vi "LED_voltage_stability.vi"() -> ()   [LabVIEW 2012]
uses:
  <instrlib>/Keithley 2600 Series/Public/Channel.ctl
  <vilib>/Utility/file.llb/Read From Spreadsheet File (DBL).vi
  <vilib>/Utility/file.llb/Write To Spreadsheet File (string).vi
  <vilib>/Utility/file.llb/Write To Spreadsheet File (DBL).vi
  <instrlib>/Keithley 2600 Series/Keithley 2600 Series.lvlib
  <vilib>/Analysis/NI_AALPro.lvlib
  <vilib>/gmath/NI_Gmath.lvlib
panel:
  out "CurDen array":string[](array[string])
  out "power array":string[](array[string])
  out "Power(W)":dbl
  out "DeltaWL":dbl[](array[numeric])
  out "data path":path
  out "DarkSpectrum path":path
  out "Info path":path
  out "AllSpectrum path":path
  out "EQE array":string[](array[string])
  out "LPE array":string[](array[string])
  out "CE array":string[](array[string])
  out "L/L0 array":string[](array[string])
  out "Lum array":string[](array[string])
  out "voltage array":string[](array[string])
  out "current array":string[](array[string])
  out "time array":string[](array[string])
  out "Info3":string
  out "Info2":string
  out "Info1":string
  out "time string":string
  out "date string":string
  out "Status":string
  in  "Tab Control":T1(tab)
  in  "VISA resource name":refnum<visa-resource-name>
  in  "Source Voltage (V)":dbl=2.5 format="%#_5f"
  in  "Current Limit (A)":dbl=1.0 format="%#_5e"
  in  "Integration Time (ms)":dbl=10.0
  in  "Interval (s)":u32=5
  in  "Initial wait (ms)":u32=2000
  in  "Calibration File":path
  in  "Dev_Area (m2)":dbl=3e-06
  in  "WL_high":dbl=785.0
  in  "WL_low":dbl=365.0
  in  "Ratio for auto stop":dbl
  in  "File Path":path
  in  "Auto stop":bool
  in  "Boxcar Width":i32
  in  "Sample description:":string="Please write here..."
  out "Measured Voltage (V)":string
  out "Measured Current (A)":string
  out "WL_2":dbl format="%#_5g"
  out "WL_1":dbl format="%#_5g"
  out "EQE (%)":dbl format="%_3e"
  out "Lum. Pow. Eff. (lm/W)":dbl format="%_3e"
  out "Lum.(cd/m2)":dbl format="%_3e"
  out "Cur. Eff. (cd/A)":dbl format="%_3e"
  out "Lum0":dbl format="%_3e"
  out "Lum/Lum0":dbl format="%_3e"
  out "Time (s)":dbl
  out "Spectra":T2(graph)
  out "Graph":cluster{dbl[], dbl[]}(graph)
  out "Measured_Current(A)":dbl format="%_3e"
  out "Measured_voltage(V)":dbl format="%_3e"
  in  "Ring":i32(ring)=1 items=["L/L0", "Lum", "C.E.", "L.P.E.", "EQE", "Power"]
  out "Maximum Intensity":i32 format="%.2e"
  out "BoxcarWidth":i32
  out "Detector Saturated":bool
  out "All Info":string
  out "VISA resource name out":refnum<visa-resource-name>
  out "error out":errorcluster
  out "x2":i32
  out "x1":i32
  out "Photon_count":dbl
  out "Energy_WL":dbl[](array[numeric])
  out "Candela":dbl
  out "Abs_Irr (W/nm)":dbl[](array[numeric])
  out "Dark_spectrum":dbl[](array[numeric])
  out "Keithley":bool
  out "Spectrometer":bool
  out "Current density (mA/cm2)":dbl
  out "Iso. Coef. itpl":dbl[](array[numeric]) format="%_6g"
  out "WL itpl":dbl[](array[numeric]) format="%_6g"
  out "EyeRespCoef.":dbl[](array[numeric])
  out "WL_EyeResp":dbl[](array[numeric])
  out "WL_cal":dbl[](array[numeric])
  out "cal_CountsToAbsIrr":dbl[](array[numeric])
  in  "Start":bool
  in  "stop":bool
  out "Measured_Spectrum":dbl[](array[numeric])
  out "Wrapper Out":u64
  out "WL_spectrometer":dbl[](array[numeric])
  out "Number of Spectrometers":i32
  out "Node Out":string
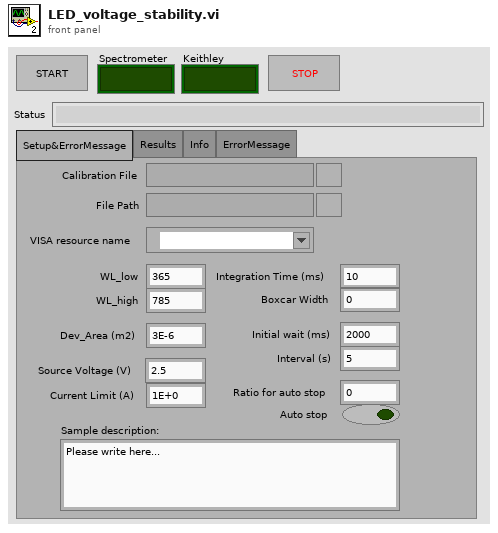
[diagram p1: front panel]
types:
  T1 = enum32{"Setup&ErrorMessage", "Results", "Info", "ErrorMessage"}
  T2 = cluster{"WL_spectrometer":dbl[], "Dark_spectrum":dbl[]}
  T3 = enum32{"Current", "Voltage", "IV", "Resistance", "Power"}
  T4 = typedef "Keithley 2600 Series.lvlib/Channel.ctl" = enum32{"Channel A", "Channel B"}
  T5 = cluster{"WL_spectrometer":dbl[], "Measured_Spectrum":dbl[]}
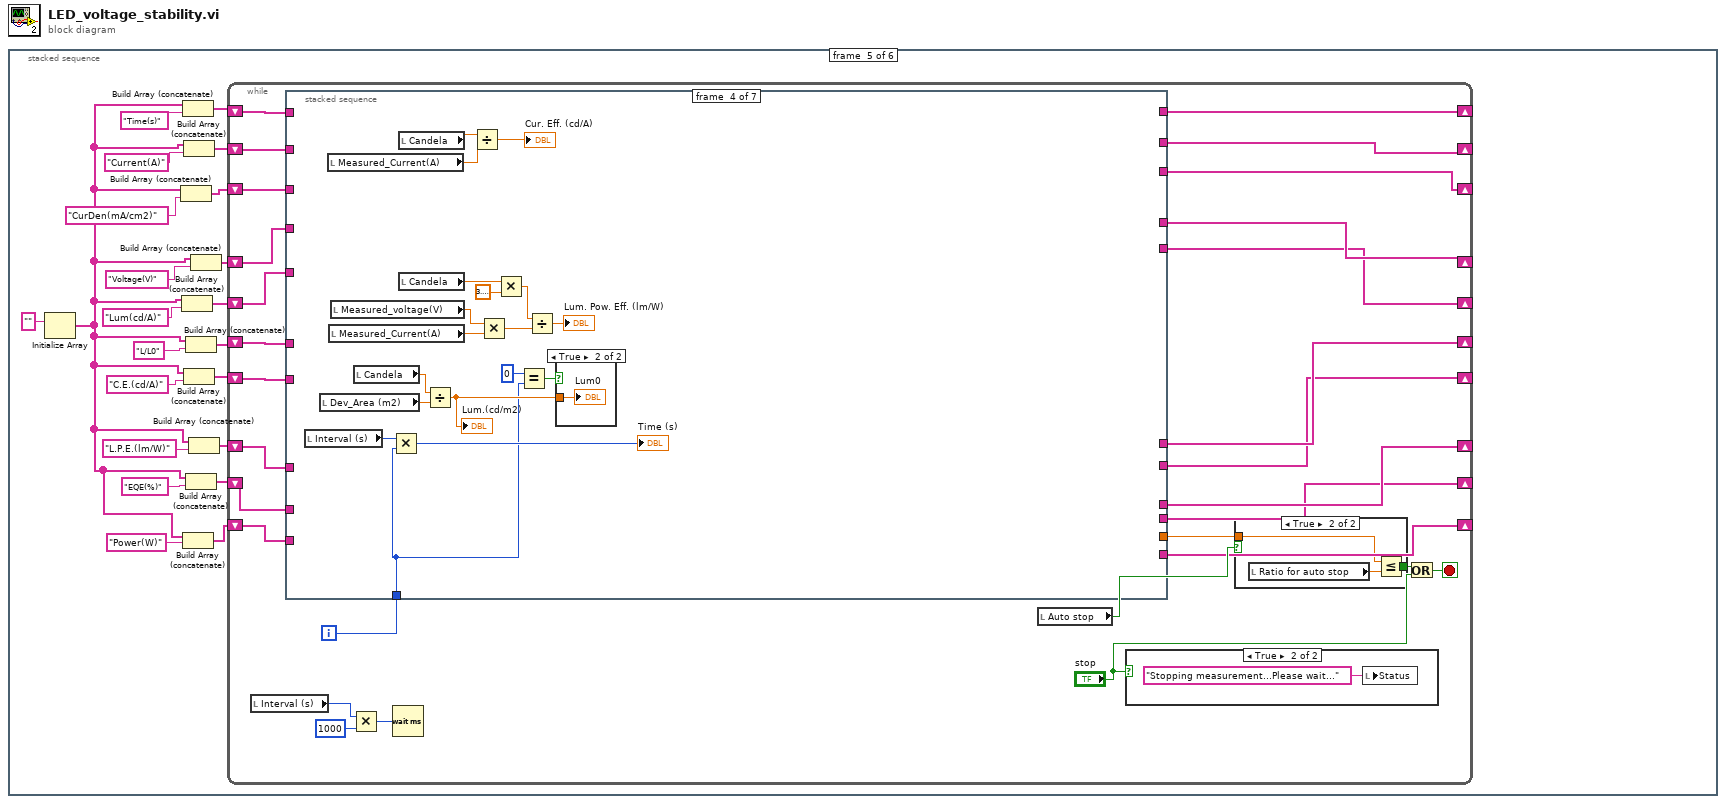
[diagram p0: block diagram]
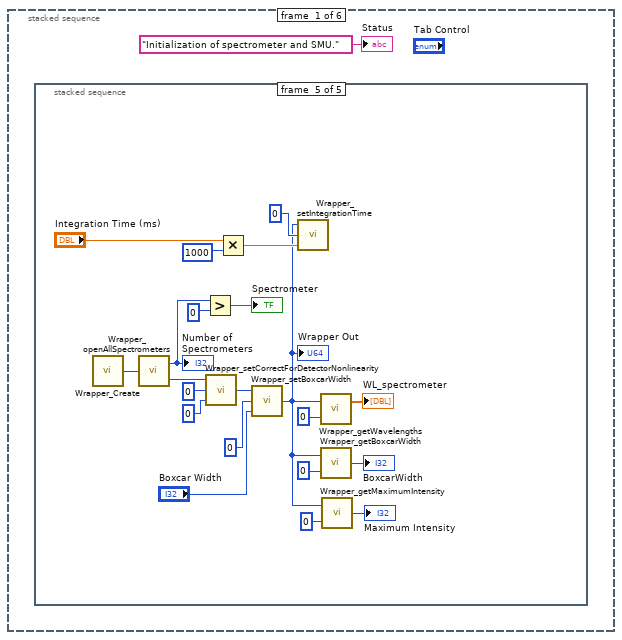
[diagram p2: hidden frame]
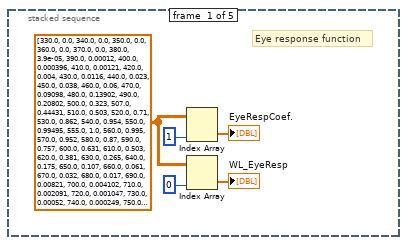
[diagram p3: hidden frame]
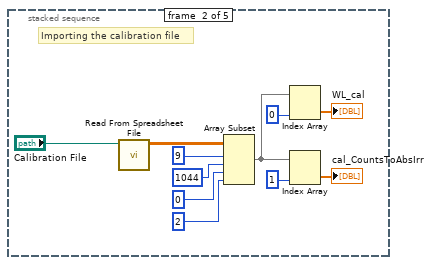
[diagram p4: hidden frame]
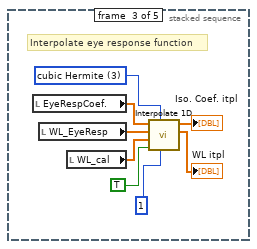
[diagram p5: hidden frame]
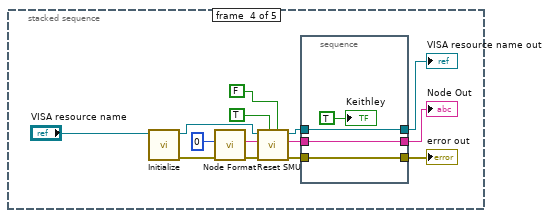
[diagram p6: hidden frame]
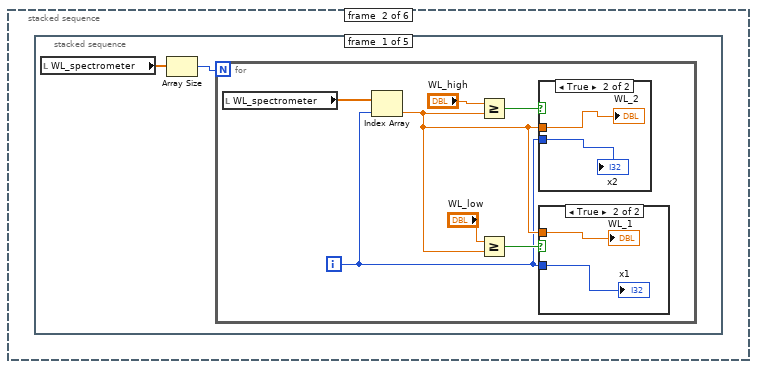
[diagram p7: hidden frame]
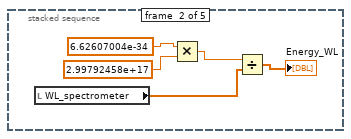
[diagram p10: hidden frame]
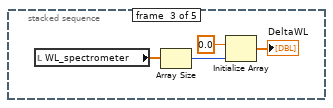
[diagram p11: hidden frame]
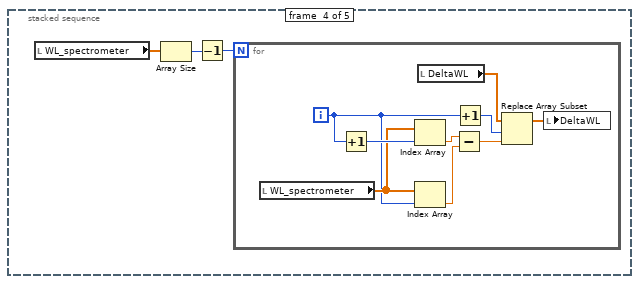
[diagram p12: hidden frame]
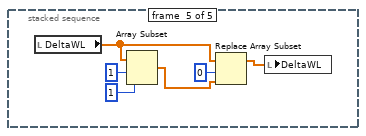
[diagram p13: hidden frame]
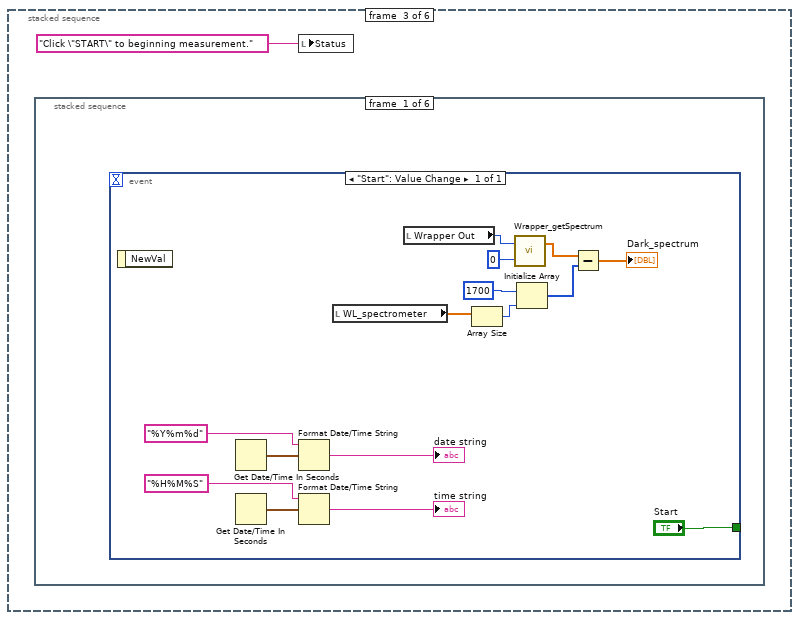
[diagram p14: hidden frame]
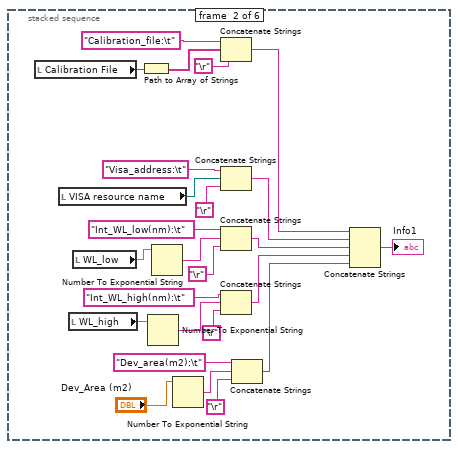
[diagram p15: hidden frame]
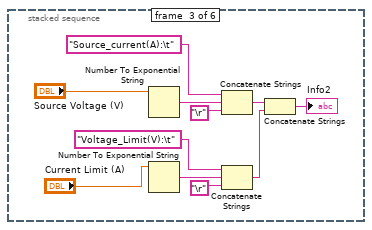
[diagram p16: hidden frame]
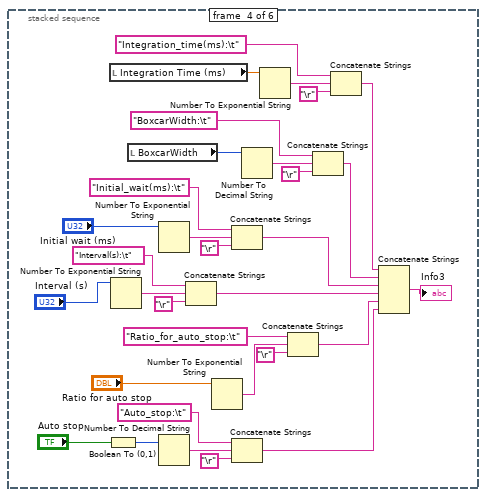
[diagram p17: hidden frame]
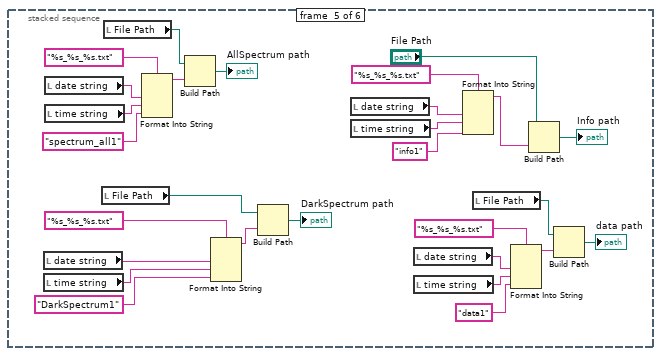
[diagram p18: hidden frame]
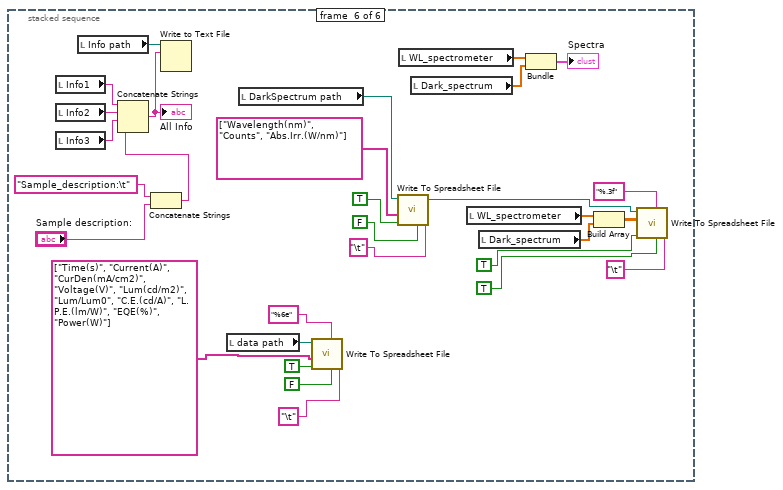
[diagram p19: hidden frame]
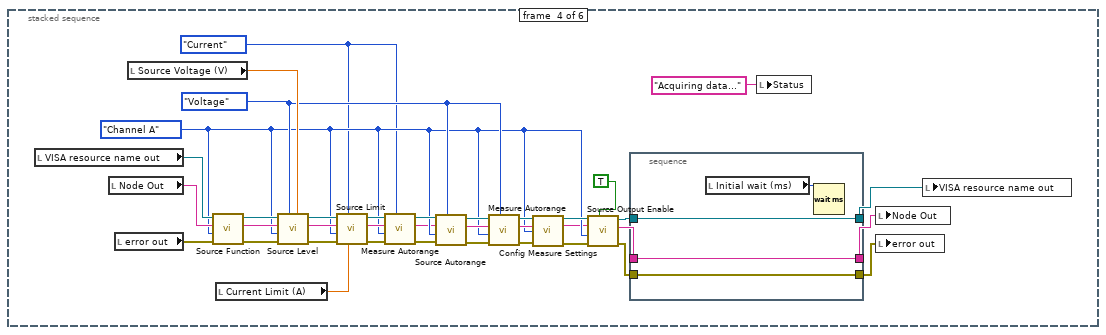
[diagram p20: hidden frame]
diagram:
  n1 = stacked-sequence {
    frame #0 {
      n2 = stacked-sequence {
        frame #0 {
          w5 = dbl[][] [[330.0, 0.0], [340.0, 0.0], [350.0, 0.0], [360.0, 0.0], [370.0, 0.0], [380.0, 3.9e-05], [390.0, 0.00012], [400.0, 0.000396], [410.0, 0.00121], [420.0, 0.004], [430.0, 0.0116], [440.0, 0.023], [450.0, 0.038], [460.0, 0.06], [470.0, 0.09098], [480.0, 0.13902], [490.0, 0.20802], [500.0, 0.323], [507.0, 0.44431], [510.0, 0.503], [520.0, 0.71], [530.0, 0.862], [540.0, 0.954], [550.0, 0.99495], [555.0, 1.0], [560.0, 0.995], [570.0, 0.952], [580.0, 0.87], [590.0, 0.757], [600.0, 0.631], [610.0, 0.503], [620.0, 0.381], [630.0, 0.265], [640.0, 0.175], [650.0, 0.107], [660.0, 0.061], [670.0, 0.032], [680.0, 0.017], [690.0, 0.00821], [700.0, 0.004102], [710.0, 0.002091], [720.0, 0.001047], [730.0, 0.00052], [740.0, 0.000249], [750.0, 0.00012], [760.0, 6e-05], [770.0, 3e-05], [780.0, 0.0], [790.0, 0.0], [800.0, 0.0], [810.0, 0.0], [820.0, 0.0], [830.0, 0.0], [840.0, 0.0], [850.0, 0.0], [860.0, 0.0], [870.0, 0.0], [880.0, 0.0], [890.0, 0.0], [900.0, 0.0], [910.0, 0.0], [920.0, 0.0], [930.0, 0.0], [940.0, 0.0], [950.0, 0.0], [960.0, 0.0], [970.0, 0.0], [980.0, 0.0], [990.0, 0.0], [1000.0, 0.0], [1010.0, 0.0], [1020.0, 0.0], [1030.0, 0.0], [1040.0, 0.0], [1050.0, 0.0], [1060.0, 0.0], [1070.0, 0.0], [1080.0, 0.0], [1090.0, 0.0], [1100.0, 0.0], [1110.0, 0.0], [1120.0, 0.0], [1130.0, 0.0], [1140.0, 0.0]] ("all rows")
          # "Eye response function"
          n3 = Index Array(array=w5, index (col)=1 ("disabled index (col)")) -> (element=→"EyeRespCoef.":dbl[])  [unwired: 1 in]
          n4 = Index Array(array=w5, index (col)=0 ("disabled index (col)")) -> (element=→"WL_EyeResp":dbl[])  [unwired: 1 in]
        }
        frame #1 {
          # "Importing the calibration file"
          n5 = call-poly <vilib>:"Read From Spreadsheet File.vi"("file path (dialog if empty)"="Calibration File") -> ("all rows"=w10:dbl[][])  [unwired: 6 in, 4 out]
          n6 = Array Subset(array=w10, index (row)=9 ("index"), length (row)=1044 ("length"), index (col)=0 ("index"), length (col)=2 ("length")) -> (w13:dbl[][])
          n7 = Index Array(array=w13, index (col)=0 ("index")) -> (element=→"WL_cal":dbl[])  [unwired: 1 in]
          n8 = Index Array(array=w13, index (col)=1 ("length")) -> (element=→"cal_CountsToAbsIrr":dbl[])  [unwired: 1 in]
        }
        frame #2 {
          w21 = 3 items=["nearest", "linear", "spline", "cubic Hermite", "Lagrange"] ("method")
          # "Interpolate eye response function"
          n9 = local read "EyeRespCoef."() -> (w24:dbl[])
          n10 = local read "WL_EyeResp"() -> (w25:dbl[])
          n11 = local read "WL_cal"() -> (w23:dbl[])
          n12 = call <vilib>:"Interpolate 1D.vi"("ntimes"=1, "method"=w21, "X is monotonic"=TRUE, "xi"=w23, "X"=w25, "Y"=w24) -> ("xi used"=→"WL itpl":dbl[], "yi"=→"Iso. Coef. itpl":dbl[])  [unwired: 3 in, 1 out]
        }
        frame #3 {
          n13 = call <instrlib>:"Initialize.vi"("VISA resource name"="VISA resource name") -> ("error out"=w37:errorcluster, "VISA resource name out"=w39:refnum<visa-resource-name>)  [unwired: 5 in, 4 out]
          n14 = call <instrlib>:"Node Format.vi"("error in"=w37, "Node (0-64)"=i8 0) -> ("error out"=w36:errorcluster, "Formatted Node"=w38:string)  [unwired: 8 out]
          n15 = call <instrlib>:"Reset SMU.vi"("SMU B (No)"=FALSE, "SMU A (No)"=TRUE, "error in (no error)"=w36, "Node In"=w38, "VISA resource name"=w39) -> ("error out"=w31:errorcluster, "Node Out"=w29:string, "VISA resource name out"=w27:refnum<visa-resource-name>)  [unwired: 4 out]
          n16 = stacked-sequence {
            tunnel: [w42] -> w30
            tunnel: w31 -> [w42]
            tunnel: w29 -> [w41]
            tunnel: [w41] -> w28
            tunnel: w27 -> [w40]
            tunnel: [w40] -> w26
            frame #0 {
              "Keithley" <- TRUE ("Keithley")
            }
          }
          "Node Out" <- w28
          "error out" <- w30
          "VISA resource name out" <- w26
        }
        frame #4 {
          n17 = call "Wrapper_Create.vi"() -> ("Wrapper"=w64:u64)
          n18 = call "Wrapper_openAllSpectrometers.vi"("Wrapper In"=w64) -> ("Number of Spectrometers"=w57:i32, "Wrapper Out"=w48:u64)
          "Number of Spectrometers" <- w57
          n19 = Greater?(x=w57, y=0) -> (0:→"Spectrometer":bool)
          n20 = call "Wrapper_setCorrectForDetectorNonlinearity.vi"("On/Off"=0, "Index"=0, "Wrapper In"=w48) -> ("Wrapper Out"=w53:u64)
          n21 = Multiply(x="Integration Time (ms)", y=1000) -> (x*y=w60:dbl)
          n22 = call "Wrapper_setBoxcarWidth.vi"("Boxcar Width"="Boxcar Width", "Index"=0, "Wrapper In"=w53) -> ("Wrapper Out"=w47:u64)
          "Wrapper Out" <- w47
          n23 = call "Wrapper_setIntegrationTime.vi"("Integration Time"=w60, "Index"=0, "Wrapper In"=w47) -> ()  [unwired: 1 out]
          n24 = call "Wrapper_getWavelengths.vi"("Index"=0, "Wrapper"=w47) -> ("WL Values"=→"WL_spectrometer":dbl[])  [unwired: 1 out]
          n25 = call "Wrapper_getBoxcarWidth.vi"("Index"=0, "Wrapper"=w47) -> ("BoxcarWidth"=→"BoxcarWidth":i32)
          n26 = call "Wrapper_getMaximumIntensity.vi"("Index"=0, "Wrapper"=w47) -> ("Maximum Intensity"=→"Maximum Intensity":i32)
        }
      }
      "Status" <- "Initialization of spectrometer and SMU." ("Measured Current (A) 2")
    }
    frame #1 {
      n27 = stacked-sequence {
        frame #0 {
          n28 = local read "WL_spectrometer"() -> (w65:dbl[])
          n29 = Array Size(array=w65) -> (size(s)=w66:i32)
          n30 = for {
            N: w66 -> [_]
            i -> [w67]
            n31 = local read "WL_spectrometer"() -> (w69:dbl[])
            n32 = Index Array(array=w69, index=w67) -> (element=w68:dbl)
            n33 = Greater Or Equal?(x="WL_high", y=w68) -> (x >= y?=w71:bool)
            n34 = Greater Or Equal?(x="WL_low", y=w68) -> (x >= y?=w70:bool)
            n35 = case shown="True" w71 {
              tunnel: w68 -> [_ w76]
              tunnel: w67 -> [_ w77]
              frame False {
              }
              frame True {
                "WL_2" <- w76
                "x2" <- w77
              }
            }
            n36 = case shown="True" w70 {
              tunnel: w68 -> [_ w74]
              tunnel: w67 -> [_ w75]
              frame False {
              }
              frame True {
                "WL_1" <- w74
                "x1" <- w75
              }
            }
          }
        }
        frame #1 {
          n37 = local read "WL_spectrometer"() -> (w81:dbl[])
          n38 = Multiply(x=6.62607004e-34, y=2.99792458e+17) -> (x*y=w80:dbl)
          n39 = Divide(x=w80, y=w81) -> (x/y=→"Energy_WL":dbl[])
        }
        frame #2 {
          n40 = local read "WL_spectrometer"() -> (w86:dbl[])
          n41 = Array Size(array=w86) -> (size(s)=w84:i32)
          n42 = Initialize Array(0.0, w84) -> (→"DeltaWL":dbl[])
        }
        frame #3 {
          n43 = local read "WL_spectrometer"() -> (w89:dbl[])
          n44 = Array Size(array=w89) -> (size(s)=w88:i32)
          n45 = Decrement(x=w88) -> (x-1=w87:i32)
          n46 = for {
            N: w87 -> [_]
            i -> [w94]
            n47 = local read "WL_spectrometer"() -> (w97:dbl[])
            n48 = Increment(x=w94) -> (x+1=w98:i32)
            n49 = Index Array(array=w97, index=w98) -> (element=w96:dbl)
            n50 = Index Array(array=w97, index=w94) -> (element=w95:dbl)
            n51 = local read "DeltaWL"() -> (w91:dbl[])
            n52 = Subtract(x=w96, y=w95) -> (x-y=w92:dbl)
            n53 = Increment(x=w94) -> (x+1=w93:i32)
            n54 = Replace Array Subset(array=w91, new element=w92, index=w93) -> (w90:dbl[])
            n55 = local write "DeltaWL"(w90) -> ()
          }
        }
        frame #4 {
          n56 = local read "DeltaWL"() -> (w99:dbl[])
          n57 = Array Subset(array=w99, index=1, length=1) -> (w100:dbl[])
          n58 = Replace Array Subset(array=w99, new element=w100, index=0) -> (w104:dbl[])
          n59 = local write "DeltaWL"(w104) -> ()
        }
      }
    }
    frame #2 {
      n60 = stacked-sequence {
        frame #0 {
          n61 = event shown="[0] \"Start\": Value Change" {
            selector: _ -> [_]
            dyn-events: _ -> [_]
            timeout: _ -> [_]
            tunnel: ["Start"] -> _
            event "Start": Value Change {
              n62 = event-data() -> ()  [unwired: 1 in, 1 out]
              n63 = Get Date/Time In Seconds() -> (seconds since 1Jan1904=w118:timestamp)
              n64 = Get Date/Time In Seconds() -> (seconds since 1Jan1904=w116:timestamp)
              n65 = Format Date/Time String(time format string (%c)="%Y%m%d" ("Timestamp string format i%cj"), seconds (now)=w118) -> (date/time string=→"date string":string)  [unwired: 1 out]
              n66 = Format Date/Time String(time format string (%c)="%H%M%S" ("Timestamp string format i%cj"), seconds (now)=w116) -> (date/time string=→"time string":string)  [unwired: 1 out]
              n67 = local read "WL_spectrometer"() -> (w111:dbl[])
              n68 = local read "Wrapper Out"() -> (w112:u64)
              n69 = Array Size(array=w111) -> (size(s)=w110:i32)
              n70 = call "Wrapper_getSpectrum.vi"("Index"=0, "Wrapper"=w112) -> ("Spectrum Values"=w108:dbl[])  [unwired: 1 out]
              n71 = Initialize Array(1700, w110) -> (w107:i32[])
              n72 = Subtract(x=w108, y=w107) -> (x-y=→"Dark_spectrum":dbl[])
            }
          }
        }
        frame #1 {
          n73 = local read "Calibration File"() -> (w122:path)
          n74 = local read "VISA resource name"() -> (w128:refnum<visa-resource-name>)
          n75 = local read "WL_high"() -> (w124:dbl)
          n76 = local read "WL_low"() -> (w123:dbl)
          n77 = Path to Array of Strings(0:w122) -> (2:w126:string[])  [unwired: 1 out]
          n78 = Number To Exponential String(number=w124) -> (E-format string=w132:string)  [unwired: 3 in]
          n79 = Number To Exponential String(number=w123) -> (E-format string=w129:string)  [unwired: 3 in]
          n80 = Number To Exponential String(number="Dev_Area (m2)") -> (E-format string=w135:string)  [unwired: 3 in]
          n81 = Concatenate Strings("Calibration_file:\t" ("string"), w126, "\r") -> (w136:string)
          n82 = Concatenate Strings("Visa_address:\t" ("string"), w128, "\r") -> (w137:string)
          n83 = Concatenate Strings("Int_WL_low(nm):\t" ("string"), w129, "\r") -> (w138:string)
          n84 = Concatenate Strings("Int_WL_high(nm):\t" ("string"), w132, "\r") -> (w139:string)
          n85 = Concatenate Strings("Dev_area(m2):\t" ("string"), w135, "\r") -> (w140:string)
          n86 = Concatenate Strings(w136, w137, w138, w139, w140) -> (→"Info1":string)
        }
        frame #2 {
          n87 = Number To Exponential String(number="Source Voltage (V)") -> (E-format string=w148:string)  [unwired: 3 in]
          n88 = Number To Exponential String(number="Current Limit (A)") -> (E-format string=w151:string)  [unwired: 3 in]
          n89 = Concatenate Strings("Source_current(A):\t" ("string"), w148, "\r") -> (w153:string)
          n90 = Concatenate Strings("Voltage_Limit(V):\t" ("string"), w151, "\r") -> (w154:string)
          n91 = Concatenate Strings(w153, w154) -> (→"Info2":string)
        }
        frame #3 {
          n92 = Boolean To (0,1)(Boolean="Auto stop") -> (0, 1=w165:i16)
          n93 = local read "Integration Time (ms)"() -> (w176:dbl)
          n94 = Number To Exponential String(number="Interval (s)") -> (E-format string=w182:string)  [unwired: 3 in]
          n95 = local read "BoxcarWidth"() -> (w158:i32)
          n96 = Number To Exponential String(number="Initial wait (ms)") -> (E-format string=w178:string)  [unwired: 3 in]
          n97 = Number To Decimal String(number=w165) -> (decimal integer string=w164:string)  [unwired: 1 in]
          n98 = Concatenate Strings("Interval(s):\t" ("string"), w182, "\r") -> (w187:string)
          n99 = Number To Exponential String(number="Ratio for auto stop") -> (E-format string=w183:string)  [unwired: 3 in]
          n100 = Concatenate Strings("Initial_wait(ms):\t" ("string"), w178, "\r") -> (w186:string)
          n101 = Concatenate Strings("Auto_stop:\t" ("string"), w164, "\r") -> (w163:string)
          n102 = Number To Decimal String(number=w158) -> (decimal integer string=w162:string)  [unwired: 1 in]
          n103 = Number To Exponential String(number=w176) -> (E-format string=w175:string)  [unwired: 3 in]
          n104 = Concatenate Strings("Ratio_for_auto_stop:\t" ("string"), w183, "\r") -> (w188:string)
          n105 = Concatenate Strings("BoxcarWidth:\t" ("string"), w162, "\r") -> (w160:string)
          n106 = Concatenate Strings("Integration_time(ms):\t" ("string"), w175, "\r") -> (w159:string)
          n107 = Concatenate Strings(w159, w160, w186, w187, w188, w163) -> (→"Info3":string)
        }
        frame #4 {
          n108 = local read "date string"() -> (w202:string)
          n109 = local read "time string"() -> (w203:string)
          n110 = local read "date string"() -> (w213:string)
          n111 = local read "time string"() -> (w214:string)
          n112 = local read "File Path"() -> (w201:path)
          n113 = local read "File Path"() -> (w215:path)
          n114 = Format Into String(format string="%s_%s_%s.txt" ("Format string"), w213, w214, "spectrum_all1" ("input 2")) -> (resulting string=w212:string)  [unwired: 2 in, 1 out]
          n115 = Build Path(base path=w215, name or relative path=w212) -> (appended path=→"AllSpectrum path":path)
          n116 = Format Into String(format string="%s_%s_%s.txt" ("Format string"), w202, w203, "DarkSpectrum1" ("input 2")) -> (resulting string=w200:string)  [unwired: 2 in, 1 out]
          n117 = Build Path(base path=w201, name or relative path=w200) -> (appended path=→"DarkSpectrum path":path)
          n118 = local read "date string"() -> (w206:string)
          n119 = local read "time string"() -> (w208:string)
          n120 = local read "date string"() -> (w191:string)
          n121 = local read "time string"() -> (w192:string)
          n122 = Format Into String(format string="%s_%s_%s.txt" ("Format string"), w206, w208, "info1" ("input 2")) -> (resulting string=w209:string)  [unwired: 2 in, 1 out]
          n123 = local read "File Path"() -> (w194:path)
          n124 = Format Into String(format string="%s_%s_%s.txt" ("Format string"), w191, w192, "data1" ("input 2")) -> (resulting string=w190:string)  [unwired: 2 in, 1 out]
          n125 = Build Path(base path="File Path", name or relative path=w209) -> (appended path=→"Info path":path)
          n126 = Build Path(base path=w194, name or relative path=w190) -> (appended path=→"data path":path)
        }
        frame #5 {
          n127 = local read "Info1"() -> (w245:string)
          n128 = local read "Info2"() -> (w244:string)
          n129 = local read "Info3"() -> (w243:string)
          n130 = local read "Info path"() -> (w232:path)
          n131 = Concatenate Strings("Sample_description:\t" ("string"), "Sample description:") -> (w217:string)
          n132 = Concatenate Strings(w245, w244, w243, w217) -> (w246:string)
          "All Info" <- w246
          n133 = Write to Text File(file (use dialog)=w232, text=w246) -> ()  [unwired: 2 in, 3 out]
          n134 = local read "data path"() -> (w225:path)
          n135 = local read "DarkSpectrum path"() -> (w227:path)
          n136 = call-poly <vilib>:"Write To Spreadsheet File.vi"("delimiter (\\t)"="\t" ("delimiter (\\t)"), "transpose? (no:F)"=FALSE, "format (%s)"="%6e" ("format (%.3f)"), "append to file? (new file:F)"=TRUE, "1D data"=string[] ["Time(s)", "Current(A)", "CurDen(mA/cm2)", "Voltage(V)", "Lum(cd/m2)", "Lum/Lum0", "C.E.(cd/A)", "L.P.E.(lm/W)", "EQE(%)", "Power(W)"], "file path (dialog if empty)"=w225) -> ()  [unwired: 1 in, 2 out]
          n137 = call-poly <vilib>:"Write To Spreadsheet File.vi"("delimiter (\\t)"="\t" ("delimiter (\\t)"), "transpose? (no:F)"=FALSE, "append to file? (new file:F)"=TRUE, "1D data"=string[] ["Wavelength(nm)", "Counts", "Abs.Irr.(W/nm)"], "file path (dialog if empty)"=w227) -> ("new file path (Not A Path if cancelled)"=w226:path)  [unwired: 2 in, 1 out]
          n138 = local read "WL_spectrometer"() -> (w233:dbl[])
          n139 = local read "Dark_spectrum"() -> (w234:dbl[])
          n140 = local read "WL_spectrometer"() -> (w237:dbl[])
          n141 = local read "Dark_spectrum"() -> (w236:dbl[])
          n142 = Bundle("WL_spectrometer"=w233, "Dark_spectrum"=w234) -> (→"Spectra":T2)  [unwired: 1 in]
          n143 = Build Array(w237, w236) -> (w238:dbl[][])
          n144 = call-poly <vilib>:"Write To Spreadsheet File.vi"("delimiter (\\t)"="\t" ("delimiter (\\t)"), "transpose? (no:F)"=TRUE, "format (%.3f)"="%.3f", "append to file? (new file:F)"=TRUE, "2D data"=w238, "file path (dialog if empty)"=w226) -> ()  [unwired: 1 in, 2 out]
        }
      }
      n145 = local write "Status"("Click \"START\" to beginning measurement." ("Status")) -> ()
    }
    frame #3 {
      w250 = enum32{"Current", "Voltage"}."Current" ("Function (Current)")
      w256 = enum32{"Current", "Voltage"}."Voltage" ("Function (Current)")
      w251 = Channel."Channel A" ("Channel (Channel A)")
      n146 = local read "VISA resource name out"() -> (w275:refnum<visa-resource-name>)
      n147 = local read "Node Out"() -> (w276:string)
      n148 = local read "error out"() -> (w277:errorcluster)
      n149 = local read "Source Voltage (V)"() -> (w267:dbl)
      n150 = call <instrlib>:"Source Function.vi"("error in (no error)"=w277, "Channel (Channel A)"=w251, "Node In"=w276, "VISA resource name"=w275) -> ("error out"=w280:errorcluster, "Node Out"=w278:string, "VISA resource name out"=w279:refnum<visa-resource-name>)  [unwired: 1 in, 4 out]
      n151 = local read "Current Limit (A)"() -> (w266:dbl)
      n152 = call <instrlib>:"Source Level.vi"("Level (0.000)"=w267, "Function (Current)"=w256, "error in (no error)"=w280, "Channel (Channel A)"=w251, "Node In"=w278, "VISA resource name"=w279) -> ("error out"=w281:errorcluster, "Node Out"=w283:string, "VISA resource name out"=w282:refnum<visa-resource-name>)  [unwired: 3 out]
      n153 = call <instrlib>:"Source Limit.vi"("Limit (0.000)"=w266, "Function (Current)"=w250, "error in (no error)"=w281, "Channel (Channel A)"=w251, "Node In"=w283, "VISA resource name"=w282) -> ("error out"=w259:errorcluster, "Node Out"=w258:string, "VISA resource name out"=w257:refnum<visa-resource-name>)  [unwired: 3 out]
      n154 = call <instrlib>:"Measure Autorange.vi"("Function (Current)"=w250, "error in (no error)"=w259, "Channel (Channel A)"=w251, "Node In"=w258, "VISA resource name"=w257) -> ("error out"=w255:errorcluster, "Node Out"=w249:string, "VISA resource name out"=w254:refnum<visa-resource-name>)  [unwired: 1 in, 3 out]
      n155 = call <instrlib>:"Source Autorange.vi"("Function (Current)"=w256, "error in (no error)"=w255, "Channel (Channel A)"=w251, "Node In"=w249, "VISA resource name"=w254) -> ("error out"=w263:errorcluster, "Node Out"=w260:string, "VISA resource name out"=w264:refnum<visa-resource-name>)  [unwired: 1 in, 3 out]
      n156 = call <instrlib>:"Measure Autorange.vi"("Function (Current)"=w256, "error in (no error)"=w263, "Channel (Channel A)"=w251, "Node In"=w260, "VISA resource name"=w264) -> ("error out"=w262:errorcluster, "Node Out"=w261:string, "VISA resource name out"=w265:refnum<visa-resource-name>)  [unwired: 1 in, 3 out]
      n157 = call <instrlib>:"Config Measure Settings.vi"("VISA resource name"=w265, "Node In"=w261, "Channel (Channel A)"=w251, "error in"=w262) -> ("VISA resource name out"=w252:refnum<visa-resource-name>, "Node Out"=w248:string, "error out"=w253:errorcluster)  [unwired: 6 in, 3 out]
      n158 = call <instrlib>:"Source Output Enable.vi"("Output (Off)"=TRUE, "error in (no error)"=w253, "Channel (Channel A)"=w251, "Node In"=w248, "VISA resource name"=w252) -> ("error out"=w273:errorcluster, "Node Out"=w272:string, "VISA resource name out"=w271:refnum<visa-resource-name>)  [unwired: 4 out]
      n159 = stacked-sequence {
        tunnel: w273 -> [w287]
        tunnel: [w287] -> w268
        tunnel: w272 -> [w286]
        tunnel: [w286] -> w269
        tunnel: w271 -> [w285]
        tunnel: [w285] -> w270
        frame #0 {
          n160 = local read "Initial wait (ms)"() -> (w284:u32)
          n161 = Wait (ms)(milliseconds to wait=w284) -> ()  [unwired: 1 out]
        }
      }
      n162 = local write "Status"("Acquiring data..." ("Status")) -> ()
      n163 = local write "Node Out"(w269) -> ()
      n164 = local write "error out"(w268) -> ()
      n165 = local write "VISA resource name out"(w270) -> ()
    }
    frame #4 {
      n166 = Initialize Array("" ("element")) -> (w290:string[])  [unwired: 1 in]
      n167 = Build Array (concatenate)(w290, "CurDen(mA/cm2)" ("Status")) -> (w288:string[])
      n168 = Build Array (concatenate)(w290, "Lum(cd/A)" ("Status")) -> (w297:string[])
      n169 = Build Array (concatenate)(w290, "Time(s)" ("Status")) -> (w294:string[])
      n170 = Build Array (concatenate)(w290, "Power(W)" ("Status")) -> (w289:string[])
      n171 = Build Array (concatenate)(w290, "Current(A)" ("Status")) -> (w295:string[])
      n172 = Build Array (concatenate)(w290, "C.E.(cd/A)" ("Status")) -> (w299:string[])
      n173 = Build Array (concatenate)(w290, "L/L0" ("Status")) -> (w298:string[])
      n174 = Build Array (concatenate)(w290, "EQE(%)" ("Status")) -> (w301:string[])
      n175 = Build Array (concatenate)(w290, "L.P.E.(lm/W)" ("Status")) -> (w300:string[])
      n176 = Build Array (concatenate)(w290, "Voltage(V)" ("Status")) -> (w296:string[])
      n177 = while {
        shift-right: [w324] -> _
        shift-left: w294 -> [w332]
        shift-right: [w323] -> _
        shift-left: w295 -> [w331]
        shift-right: [w322] -> _
        shift-left: w296 -> [w330]
        shift-right: [w321] -> _
        shift-left: w297 -> [w329]
        shift-right: [w320] -> _
        shift-left: w298 -> [w328]
        shift-right: [w319] -> _
        shift-left: w299 -> [w327]
        shift-right: [w317] -> _
        shift-left: w301 -> [w325]
        shift-right: [w318] -> _
        shift-left: w300 -> [w326]
        shift-right: [w314] -> _
        shift-left: w289 -> [w315]
        shift-right: [w312] -> _
        shift-left: w288 -> [w313]
        i -> [w336]
        stop <- w335 stop-if-true
        n178 = local read "Interval (s)"() -> (w333:u32)
        n179 = stacked-sequence {
          tunnel: w336 -> [_ _ _ w447 _ _ _]
          tunnel: w332 -> [_ _ _ _ _ _ w530]
          tunnel: w331 -> [_ _ _ _ _ _ w529]
          tunnel: w330 -> [_ _ _ _ _ _ w528]
          tunnel: w329 -> [_ _ _ _ _ _ w527]
          tunnel: w328 -> [_ _ _ _ _ _ w526]
          tunnel: w327 -> [_ _ _ _ _ _ w525]
          tunnel: w326 -> [_ _ _ _ _ _ w524]
          tunnel: w325 -> [_ _ _ _ _ _ w523]
          tunnel: [_ _ _ _ _ _ w500] -> w324
          tunnel: [_ _ _ _ _ _ w499] -> w323
          tunnel: [_ _ _ _ _ _ w497] -> w322
          tunnel: [_ _ _ _ _ _ w486] -> w321
          tunnel: [_ _ _ _ _ _ w485] -> w320
          tunnel: [_ _ _ _ _ _ w487] -> w319
          tunnel: [_ _ _ _ _ _ w488] -> w318
          tunnel: [_ _ _ _ _ _ w489] -> w317
          tunnel: w315 -> [_ _ _ _ _ _ w504]
          tunnel: [_ _ _ _ _ _ w490] -> w314
          tunnel: w313 -> [_ _ _ _ _ _ w501]
          tunnel: [_ _ _ _ _ _ w498] -> w312
          tunnel: [_ _ _ _ w466 _ _] -> w311
          frame #0 {
            w362 = Channel."Channel A" ("Channel (Channel A)")
            n180 = local read "VISA resource name out"() -> (w359:refnum<visa-resource-name>)
            n181 = local read "Node Out"() -> (w360:string)
            n182 = local read "error out"() -> (w361:errorcluster)
            n183 = local read "WL_spectrometer"() -> (w349:dbl[])
            n184 = local read "Wrapper Out"() -> (w352:u64)
            n185 = call <instrlib>:"Measure.vi"("Function (Current)"=T3."Current", "error in (no error)"=w361, "Channel (Channel A)"=w362, "Node In"=w360, "VISA resource name"=w359) -> ("error out"=w370:errorcluster, "Output"=w344:string, "Node Out"=w369:string, "VISA resource name out"=w368:refnum<visa-resource-name>)  [unwired: 2 in, 1 out]
            "Measured Current (A)" <- w344
            n186 = Array Size(array=w349) -> (size(s)=w350:i32)
            n187 = call "Wrapper_getSpectrum.vi"("Index"=0, "Wrapper"=w352) -> ("Spectrum Values"=w347:dbl[])  [unwired: 1 out]
            n188 = call <instrlib>:"Measure.vi"("Function (Current)"=T3."Voltage", "error in (no error)"=w370, "Channel (Channel A)"=w362, "Node In"=w369, "VISA resource name"=w368) -> ("error out"=w364:errorcluster, "Output"=w345:string, "Node Out"=w366:string, "VISA resource name out"=w365:refnum<visa-resource-name>)  [unwired: 2 in, 1 out]
            "Measured Voltage (V)" <- w345
            n189 = Initialize Array(1700, w350) -> (w348:i32[])
            n190 = Fract/Exp String To Number(string=w345) -> (number=→"Measured_voltage(V)":dbl)  [unwired: 3 in, 1 out]
            n191 = local write "VISA resource name out"(w365) -> ()
            n192 = local write "Node Out"(w366) -> ()
            n193 = local write "error out"(w364) -> ()
            n194 = Subtract(x=w347, y=w348) -> (x-y=→"Measured_Spectrum":dbl[])
            n195 = local read "Dev_Area (m2)"() -> (w353:dbl)
            n196 = Fract/Exp String To Number(string=w344) -> (number=w356:dbl)  [unwired: 3 in, 1 out]
            "Measured_Current(A)" <- w356
            n197 = Divide(x=w356, y=w353) -> (x/y=w357:dbl)
            n198 = Multiply(x=w357, y=0.1) -> (x*y=→"Current density (mA/cm2)":dbl)
          }
          frame #1 {
            n199 = local read "Integration Time (ms)"() -> (w411:dbl)
            n200 = local read "Measured_Spectrum"() -> (w414:dbl[])
            n201 = local read "cal_CountsToAbsIrr"() -> (w407:dbl[])
            n202 = local read "Dark_spectrum"() -> (w413:dbl[])
            n203 = local read "Measured_Spectrum"() -> (w405:dbl[])
            n204 = local read "WL_spectrometer"() -> (w404:dbl[])
            n205 = Subtract(x=w414, y=w413) -> (x-y=w408:dbl[])
            n206 = Bundle("WL_spectrometer"=w404, "Measured_Spectrum"=w405) -> (w406:T5)  [unwired: 1 in]
            n207 = local read "x2"() -> (w387:i32)
            n208 = local read "x1"() -> (w386:i32)
            n209 = local read "WL_spectrometer"() -> (w384:dbl[])
            n210 = local read "x2"() -> (w385:i32)
            n211 = local read "x1"() -> (w382:i32)
            n212 = local read "WL_spectrometer"() -> (w374:dbl[])
            n213 = Multiply(x=w411, y=0.001) -> (x*y=w412:dbl)
            n214 = local write "Spectra"(w406) -> ()
            n215 = local read "Energy_WL"() -> (w396:dbl[])
            n216 = local read "DeltaWL"() -> (w402:dbl[])
            n217 = Divide(x=w408, y=w412) -> (x/y=w409:dbl[])
            n218 = Multiply(x=w407, y=w409) -> (x*y=w403:dbl[])
            n219 = Subtract(x=w387, y=w386) -> (x-y=w392:i32)
            n220 = Subtract(x=w385, y=w382) -> (x-y=w389:i32)
            n221 = Divide(x=w403, y=w402) -> (x/y=w401:dbl[])
            n222 = Increment(x=w392) -> (x+1=w391:i32)
            n223 = Divide(x=w401, y=1000000.0) -> (x/y=w372:dbl[])
            "Abs_Irr (W/nm)" <- w372
            n224 = Increment(x=w389) -> (x+1=w388:i32)
            n225 = Divide(x=w372, y=w396) -> (x/y=w393:dbl[])
            n226 = local read "Wrapper Out"() -> (w399:u64)
            n227 = call <vilib>:"Uneven Numeric Integration.vi"("T"=w374, "X"=w372) -> ("result"=→"Power(W)":dbl)  [unwired: 8 in, 1 out]
            n228 = Array Subset(array=w393, index=w386, length=w391) -> (w390:dbl[])
            n229 = Array Subset(array=w384, index=w382, length=w388) -> (w383:dbl[])
            n230 = local read "Measured_Current(A)"() -> (w376:dbl)
            n231 = call <vilib>:"Uneven Numeric Integration.vi"("T"=w383, "X"=w390) -> ("result"=w395:dbl)  [unwired: 8 in, 1 out]
            n232 = call "Wrapper_isSaturated.vi"("Index"=0, "Wrapper"=w399) -> ("Is Saturated?"=w397:u8)
            n233 = Multiply(x=w395, y=100.0) -> (x*y=w377:dbl)
            "Photon_count" <- w377
            n234 = Divide(x=w376, y=1.60217662e-19) -> (x/y=w378:dbl)
            n235 = case shown="0, Default" w397 {
              frame 0, Default {
                "Detector Saturated" <- FALSE
              }
              frame 1 {
                n236 = local write "Detector Saturated"(TRUE ("Det.Sat.")) -> ()
              }
            }
            n237 = Divide(x=w377, y=w378) -> (x/y=w381:dbl)
            n238 = Divide(x=w381, y=3.152) -> (x/y=→"EQE (%)":dbl)
          }
          frame #2 {
            n239 = local read "Measured_Spectrum"() -> (w440:dbl[])
            n240 = local read "AllSpectrum path"() -> (w435:path)
            n241 = local read "WL_spectrometer"() -> (w441:dbl[])
            n242 = local read "Iso. Coef. itpl"() -> (w420:dbl[])
            n243 = local read "Abs_Irr (W/nm)"() -> (w419:dbl[])
            n244 = local read "WL_spectrometer"() -> (w418:dbl[])
            n245 = local read "Abs_Irr (W/nm)"() -> (w439:dbl[])
            n246 = Multiply(x=w420, y=w419) -> (x*y=w421:dbl[])
            n247 = call-poly <vilib>:"Write To Spreadsheet File.vi"("delimiter (\\t)"="\t" ("delimiter (\\t)"), "transpose? (no:F)"=FALSE, "append to file? (new file:F)"=TRUE, "1D data"=string[] ["Wavelength(nm)", "Counts", "Abs.Irr.(W/nm)"], "file path (dialog if empty)"=w435) -> ("new file path (Not A Path if cancelled)"=w433:path)  [unwired: 2 in, 1 out]
            n248 = Build Array(w441, w440, w439) -> (w442:dbl[][])
            n249 = call <vilib>:"Uneven Numeric Integration.vi"("T"=w418, "X"=w421) -> ("result"=w422:dbl)  [unwired: 8 in, 1 out]
            n250 = call-poly <vilib>:"Write To Spreadsheet File.vi"("delimiter (\\t)"="\t" ("delimiter (\\t)"), "transpose? (no:F)"=TRUE, "format (%.3f)"="%6e", "append to file? (new file:F)"=TRUE, "2D data"=w442, "file path (dialog if empty)"=w433) -> ("new file path (Not A Path if cancelled)"=w429:path)  [unwired: 1 in, 1 out]
            n251 = Multiply(x=w422, y=683.002) -> (x*y=w427:dbl)
            n252 = Multiply(x=3.141592653589793, y=3.152) -> (x*y=w423:dbl)
            n253 = Divide(x=w427, y=w423) -> (x/y=→"Candela":dbl)
            n254 = call-poly <vilib>:"Write To Spreadsheet File.vi"("delimiter (\\t)"="\t" ("delimiter (\\t)"), "transpose? (no:F)"=TRUE, "append to file? (new file:F)"=TRUE, "1D data"=string[] ["", "", "", " "], "file path (dialog if empty)"=w429) -> ()  [unwired: 2 in, 2 out]
          }
          frame #3 {
            n255 = local read "Interval (s)"() -> (w448:u32)
            n256 = local read "Dev_Area (m2)"() -> (w459:dbl)
            n257 = local read "Measured_Current(A)"() -> (w457:dbl)
            n258 = local read "Measured_Current(A)"() -> (w454:dbl)
            n259 = local read "Measured_voltage(V)"() -> (w453:dbl)
            n260 = local read "Candela"() -> (w460:dbl)
            n261 = Multiply(x=w448, y=w447) -> (x*y=→"Time (s)":u32)
            n262 = local read "Candela"() -> (w458:dbl)
            n263 = local read "Candela"() -> (w456:dbl)
            n264 = Divide(x=w460, y=w459) -> (x/y=w450:dbl)
            "Lum.(cd/m2)" <- w450
            n265 = Divide(x=w458, y=w457) -> (x/y=→"Cur. Eff. (cd/A)":dbl)
            n266 = Multiply(x=w453, y=w454) -> (x*y=w462:dbl)
            n267 = Multiply(x=w456, y=3.141592653589793) -> (x*y=w463:dbl)
            n268 = Equal?(x=0, y=w447) -> (x = y?=w451:bool)
            n269 = Divide(x=w463, y=w462) -> (x/y=→"Lum. Pow. Eff. (lm/W)":dbl)
            n270 = case shown="True" w451 {
              tunnel: w450 -> [_ w465]
              frame False {
              }
              frame True {
                "Lum0" <- w465
              }
            }
          }
          frame #4 {
            n271 = local read "Lum.(cd/m2)"() -> (w467:dbl)
            n272 = local read "Lum0"() -> (w468:dbl)
            n273 = Divide(x=w467, y=w468) -> (x/y=w466:dbl)
            "Lum/Lum0" <- w466
          }
          frame #5 {
            n274 = local read "Current density (mA/cm2)"() -> (w470:dbl)
            n275 = local read "Measured_Current(A)"() -> (w471:dbl)
            n276 = local read "Lum. Pow. Eff. (lm/W)"() -> (w476:dbl)
            n277 = local read "Measured_voltage(V)"() -> (w480:dbl)
            n278 = local read "Cur. Eff. (cd/A)"() -> (w477:dbl)
            n279 = local read "Lum.(cd/m2)"() -> (w479:dbl)
            n280 = local read "Lum/Lum0"() -> (w478:dbl)
            n281 = local read "Power(W)"() -> (w469:dbl)
            n282 = local read "Time (s)"() -> (w472:dbl)
            n283 = local read "EQE (%)"() -> (w475:dbl)
            n284 = local read "data path"() -> (w473:path)
            n285 = Build Array(w472, w471, w470, w480, w479, w478, w477, w476, w475, w469) -> (w474:dbl[])
            n286 = call-poly <vilib>:"Write To Spreadsheet File.vi"("delimiter (\\t)"="\t" ("delimiter (\\t)"), "transpose? (no:F)"=FALSE, "format (%.3f)"="%6e", "append to file? (new file:F)"=TRUE, "1D data"=w474, "file path (dialog if empty)"=w473) -> ()  [unwired: 1 in, 2 out]
          }
          frame #6 {
            n287 = local read "Lum. Pow. Eff. (lm/W)"() -> (w513:dbl)
            n288 = local read "Current density (mA/cm2)"() -> (w502:dbl)
            n289 = local read "Measured_Current(A)"() -> (w510:dbl)
            n290 = local read "Measured_voltage(V)"() -> (w509:dbl)
            n291 = local read "Cur. Eff. (cd/A)"() -> (w512:dbl)
            n292 = local read "Lum.(cd/m2)"() -> (w508:dbl)
            n293 = local read "Lum/Lum0"() -> (w507:dbl)
            n294 = local read "Power(W)"() -> (w503:dbl)
            n295 = local read "Time (s)"() -> (w511:dbl)
            n296 = local read "EQE (%)"() -> (w514:dbl)
            n297 = Number To Exponential String(number=w511) -> (E-format string=w515:string)  [unwired: 3 in]
            n298 = Number To Exponential String(number=w510) -> (E-format string=w516:string)  [unwired: 3 in]
            n299 = Number To Exponential String(number=w502) -> (E-format string=w506:string)  [unwired: 3 in]
            n300 = Number To Exponential String(number=w509) -> (E-format string=w517:string)  [unwired: 3 in]
            n301 = Number To Exponential String(number=w508) -> (E-format string=w518:string)  [unwired: 3 in]
            n302 = Number To Exponential String(number=w507) -> (E-format string=w519:string)  [unwired: 3 in]
            n303 = Number To Exponential String(number=w512) -> (E-format string=w520:string)  [unwired: 3 in]
            n304 = Number To Exponential String(number=w513) -> (E-format string=w521:string)  [unwired: 3 in]
            n305 = Number To Exponential String(number=w514) -> (E-format string=w522:string)  [unwired: 3 in]
            n306 = Number To Exponential String(number=w503) -> (E-format string=w505:string)  [unwired: 3 in]
            n307 = Build Array (concatenate)(w525, w520) -> (w487:string[])
            "CE array" <- w487
            n308 = Build Array (concatenate)(w530, w515) -> (w500:string[])
            "time array" <- w500
            n309 = Build Array (concatenate)(w529, w516) -> (w499:string[])
            "current array" <- w499
            n310 = Build Array (concatenate)(w501, w506) -> (w498:string[])
            "CurDen array" <- w498
            n311 = Build Array (concatenate)(w527, w518) -> (w486:string[])
            "Lum array" <- w486
            n312 = Build Array (concatenate)(w526, w519) -> (w485:string[])
            "L/L0 array" <- w485
            n313 = Build Array (concatenate)(w524, w521) -> (w488:string[])
            "LPE array" <- w488
            n314 = Build Array (concatenate)(w523, w522) -> (w489:string[])
            "EQE array" <- w489
            n315 = Build Array (concatenate)(w528, w517) -> (w497:string[])
            "voltage array" <- w497
            n316 = Build Array (concatenate)(w504, w505) -> (w490:string[])
            "power array" <- w490
            n317 = case shown="..0" "Ring" {
              tunnel: [w531 w532 w533 w534 w535 w536] -> w491
              tunnel: w490 -> [_ _ _ _ _ w536]
              tunnel: w489 -> [_ _ _ _ w535 _]
              tunnel: w488 -> [_ _ _ w534 _ _]
              tunnel: w487 -> [_ _ w533 _ _ _]
              tunnel: w486 -> [_ w532 _ _ _ _]
              tunnel: w485 -> [w531 _ _ _ _ _]
              frame ..0 {
              }
              frame 1 {
              }
              frame 2 {
              }
              frame 3 {
              }
              frame 4 {
              }
              frame 5.. {
              }
            }
            n318 = local read "time array"() -> (w496:string[])
            n319 = Fract/Exp String To Number(string=w496) -> (number=w494:dbl[])  [unwired: 3 in, 1 out]
            n320 = Fract/Exp String To Number(string=w491) -> (number=w495:dbl[])  [unwired: 3 in, 1 out]
            n321 = Bundle(w494, w495) -> (→"Graph":cluster{dbl[], dbl[]})  [unwired: 1 in]
          }
        }
        n322 = Multiply(x=w333, y=u32 1000) -> (x*y=w338:u32)
        n323 = Wait (ms)(milliseconds to wait=w338) -> ()  [unwired: 1 out]
        n324 = local read "Auto stop"() -> (w316:bool)
        n325 = case shown="True" "stop" {
          frame False {
          }
          frame True {
            n326 = local write "Status"("Stopping measurement...Please wait..." ("Status")) -> ()
          }
        }
        n327 = case shown="True" w316 {
          tunnel: [FALSE w343] -> w334
          tunnel: w311 -> [_ w341]
          frame False {
          }
          frame True {
            n328 = local read "Ratio for auto stop"() -> (w342:dbl)
            n329 = Less Or Equal?(x=w341, y=w342) -> (x <= y?=w343:bool)
          }
        }
        n330 = Or(x=w334, y="stop") -> (x .or. y?=w335:bool)
      }
    }
    frame #5 {
      n331 = local read "VISA resource name out"() -> (w545:refnum<visa-resource-name>)
      n332 = local read "Wrapper Out"() -> (w546:u64)
      n333 = local read "Node Out"() -> (w542:string)
      n334 = local read "error out"() -> (w543:errorcluster)
      n335 = local write "Spectrometer"(FALSE ("Spectrometer")) -> ()
      n336 = call "Wrapper_closeAllSpectrometers.vi"("Wrapper In"=w546) -> ("Wrapper Out"=w547:u64)
      n337 = local write "Detector Saturated"(FALSE ("Det.Sat.")) -> ()
      n338 = local write "Keithley"(FALSE ("Keithley")) -> ()
      n339 = call "Wrapper_Destroy.vi"("Wrapper"=w547) -> ()
      n340 = call <instrlib>:"Source Output Enable.vi"("Output (Off)"=FALSE, "error in (no error)"=w543, "Channel (Channel A)"=Channel."Channel A", "Node In"=w542, "VISA resource name"=w545) -> ("error out"=w548:errorcluster, "Node Out"=w541:string, "VISA resource name out"=w549:refnum<visa-resource-name>)  [unwired: 4 out]
      n341 = local write "Status"("Measurement completed." ("Status")) -> ()
      n342 = call <instrlib>:"Close.vi"("error in (no error)"=w548, "VISA resource name"=w549) -> ()  [unwired: 10 out]
      n343 = local write "Node Out"(w541) -> ()
    }
  }
